vi "IncrementLogCounter.vi"   [LabVIEW 2013]
uses:
  Global.vi
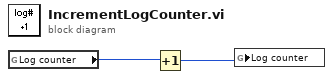
[diagram p0: block diagram]
diagram:
  n1 = global read "Global.vi" "Log counter"() -> (w2:i32)
  n2 = Increment(x=w2) -> (x+1=w1:i32)
  n3 = global write "Global.vi" "Log counter"(w1) -> ()
